vi "SquareWaveSubVI.vi"(6 "Error In":errorcluster, 8 "Frequency":dbl, 9 "DC Off":dbl, 10 "Duty Cycle":dbl, 11 "Amplitude":dbl) -> (0 "Error Out":errorcluster, 3 "Array":dbl[](array[numeric]))   [LabVIEW 2017]
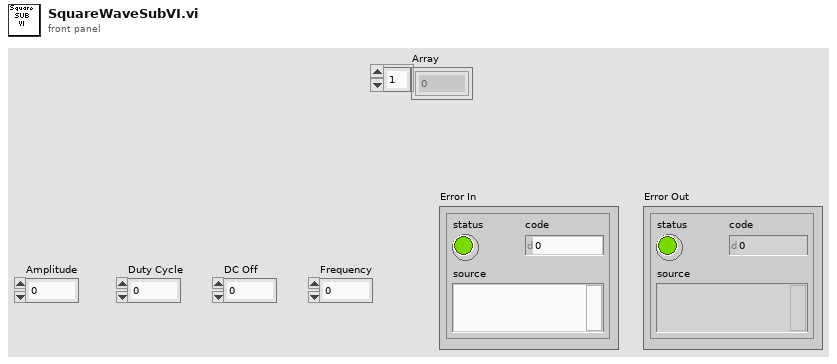
[diagram p1: front panel]
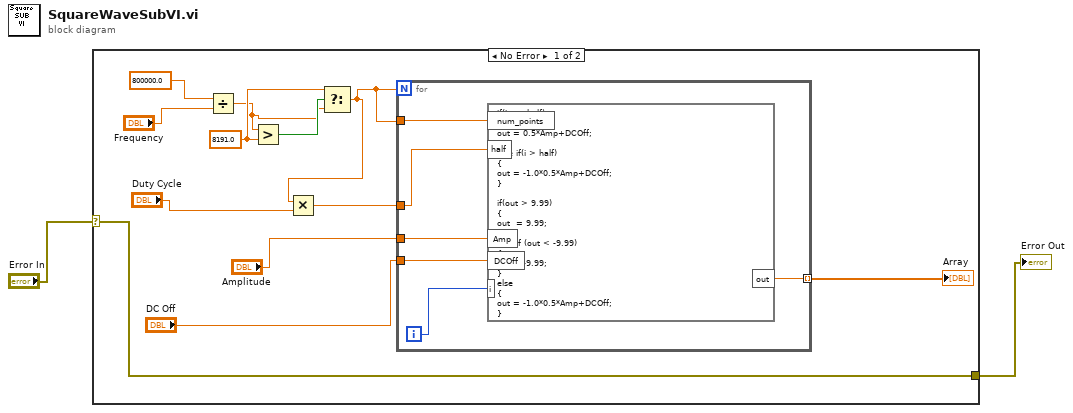
[diagram p0: block diagram]
diagram:
  n1 = case shown="No Error" "Error In" {
    selector: "Error In" -> [w14 w21]
    tunnel: [w14 w21] -> w1
    frame No Error {
      w10 = 8191.0 ("y")
      n2 = Divide(x=800000.0, y="Frequency") -> (x/y=w9:dbl)
      n3 = Greater?(x=w9, y=w10) -> (0:w11:bool)
      n4 = Select(t=w10, s=w11, f=w9) -> (s? t:f=w7:dbl)
      n5 = Multiply(x=w7, y="Duty Cycle") -> (x*y=w8:dbl)
      n6 = for {
        N: w7 -> [_]
        tunnel: w8 -> [w20]
        tunnel: w7 -> [w19]
        tunnel: "Amplitude" -> [w18]
        tunnel: "DC Off" -> [w17]
        tunnel: [w15] -> w4 mode=indexing
        i -> [w16]
        n7 = formula code="if(i <= half)\n{\nout = 0.5*Amp+DCOff;\n}\nelse if(i > half)\n{\nout = -1.0*0.5*Amp+DCOff;\n}\n\nif(out > 9.99)\n{\nout  = 9.99;\n}\nelse if (out < -9.99)\n{\nout = -9.99;\n}\nelse\n{\nout = -1.0*0.5*Amp+DCOff;\n}"("half"=w20, "num_points"=w19, "Amp"=w18, "DCOff"=w17, "i"=w16) -> ("out"=w15:dbl)
      }
      "Array" <- w4
    }
    frame Error {
    }
  }
  "Error Out" <- w1
